vi "test arr, flatten and get type&size.vi"() -> ()   [LabVIEW 2018, in "LV-Julia_ZMQ-Roundtrip_lib.lvlib"]
uses:
  LV-Julia_ZMQ-Roundtrip_lib.lvlib
  95fe096e-f04b-44d4-8552-6e65fa067250.vi
panel:
  out "sizes":i32[](array[numeric])
  out "numtype":string
  out "error out":errorcluster
  in  "Array":cdb[][][](array[numeric])
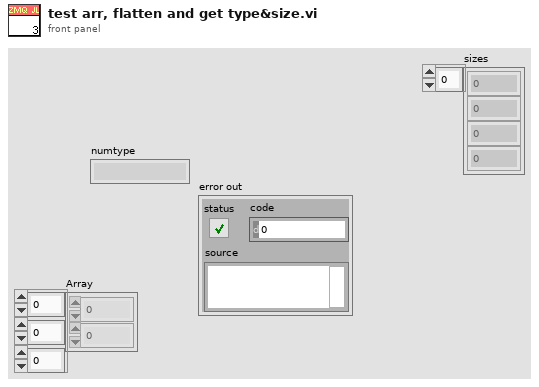
[diagram p1: front panel]
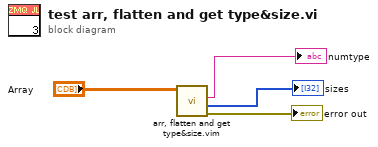
[diagram p0: block diagram]
diagram:
  n1 = call "arr, flatten and get type&size.vim"("Array in in"="Array") -> ("error out"=→"error out":errorcluster, "sizes"=→"sizes":i32[], "numtype"=→"numtype":string)  [unwired: 7 in, 1 out]
